vi "StartEqualization.vi"(8 "error in (no error)":errorcluster, 11 "reference in":refnum<class "niMmWave_Transceiver.lvclass">) -> (0 "error out":errorcluster, 2 "channel":T1, 3 "reference out":refnum<class "niMmWave_Transceiver.lvclass">)   [LabVIEW 2019, in "niMmWave_Transceiver.lvclass"]
doc: "Starts generating calibration pulse and prepares RX for acquisition"
uses:
  niMmWave_Transceiver.lvclass
  C:/Barkhausen mmWave radar/Development/LV/Barkhausen mmWave hardware control/Host/SubVIs/mmWave instrument_class/mmWave instrument.lvclass
  mmWave instrument_class/Instrument state.ctl
  Low-level/TypeDefs/TX FPGA Reference.ctl
  Low-level/TypeDefs/TX trigger config.ctl
  FPGA/SubVIs/Utility/FPGA driver trigger source.ctl
  FPGA/SubVIs/Utility/FPGA driver trigger destination.ctl
  <vilib>/Analysis/4window.llb/windowTd.ctl
  <vilib>/Analysis/1siggen.llb/Ramp Pattern by Samples.vi
  <vilib>/Analysis/2dsp.llb/Complex FFT.vi
  <vilib>/Analysis/baseanly.llb/Mean (DBL).vi
  <vilib>/Utility/error.llb/Error Cluster From Error Code.vi
  <vilib>/rvi/errors/niLvFpgaAdjustHostInterfaceError.vi
  <vilib>/measure/mascope.llb/Amplitude and Levels 1 chan.vi
  <vilib>/Analysis/0measdsp.llb/Scaled Time Domain Window (CDB).vi
  <vilib>/Analysis/6fits.llb/1D B-Spline Fit.vi
  <vilib>/rvi/interface/nirviReadWriteControl/nirviReadWriteControl.xnode
  NiFpgaLv.dll
  <vilib>/rvi/interface/Simulation/niFpgaSimulationCallBeginRW.vi
  FPGA/SubVIs/Utility/FPGA Utility.lvlib
  mmWave HW Control/mmWave HW Control.lvlib
  <vilib>/Analysis/NI_AALBase.lvlib
  <vilib>/Analysis/NI_AALPro.lvlib
  mmWave instrument_class/mmWave instrument.lvclass
  <vilib>/measure/NI_MAPro.lvlib
panel:
  out "S/N":dbl
  out "lo":dbl[](array[numeric])
  out "hi":dbl[](array[numeric])
  out "amp":dbl[](array[numeric])
  out "magnitude":T2(graph)
  out "phase":T2(graph)
  out "Waveform Graph - Dark":dbl[][](graph)
  out "phase raw":cluster{"Ramp Pattern":dbl[], dbl[]}[](graph)
  out "magnitude raw":cluster{"Ramp Pattern":dbl[], dbl[]}[](graph)
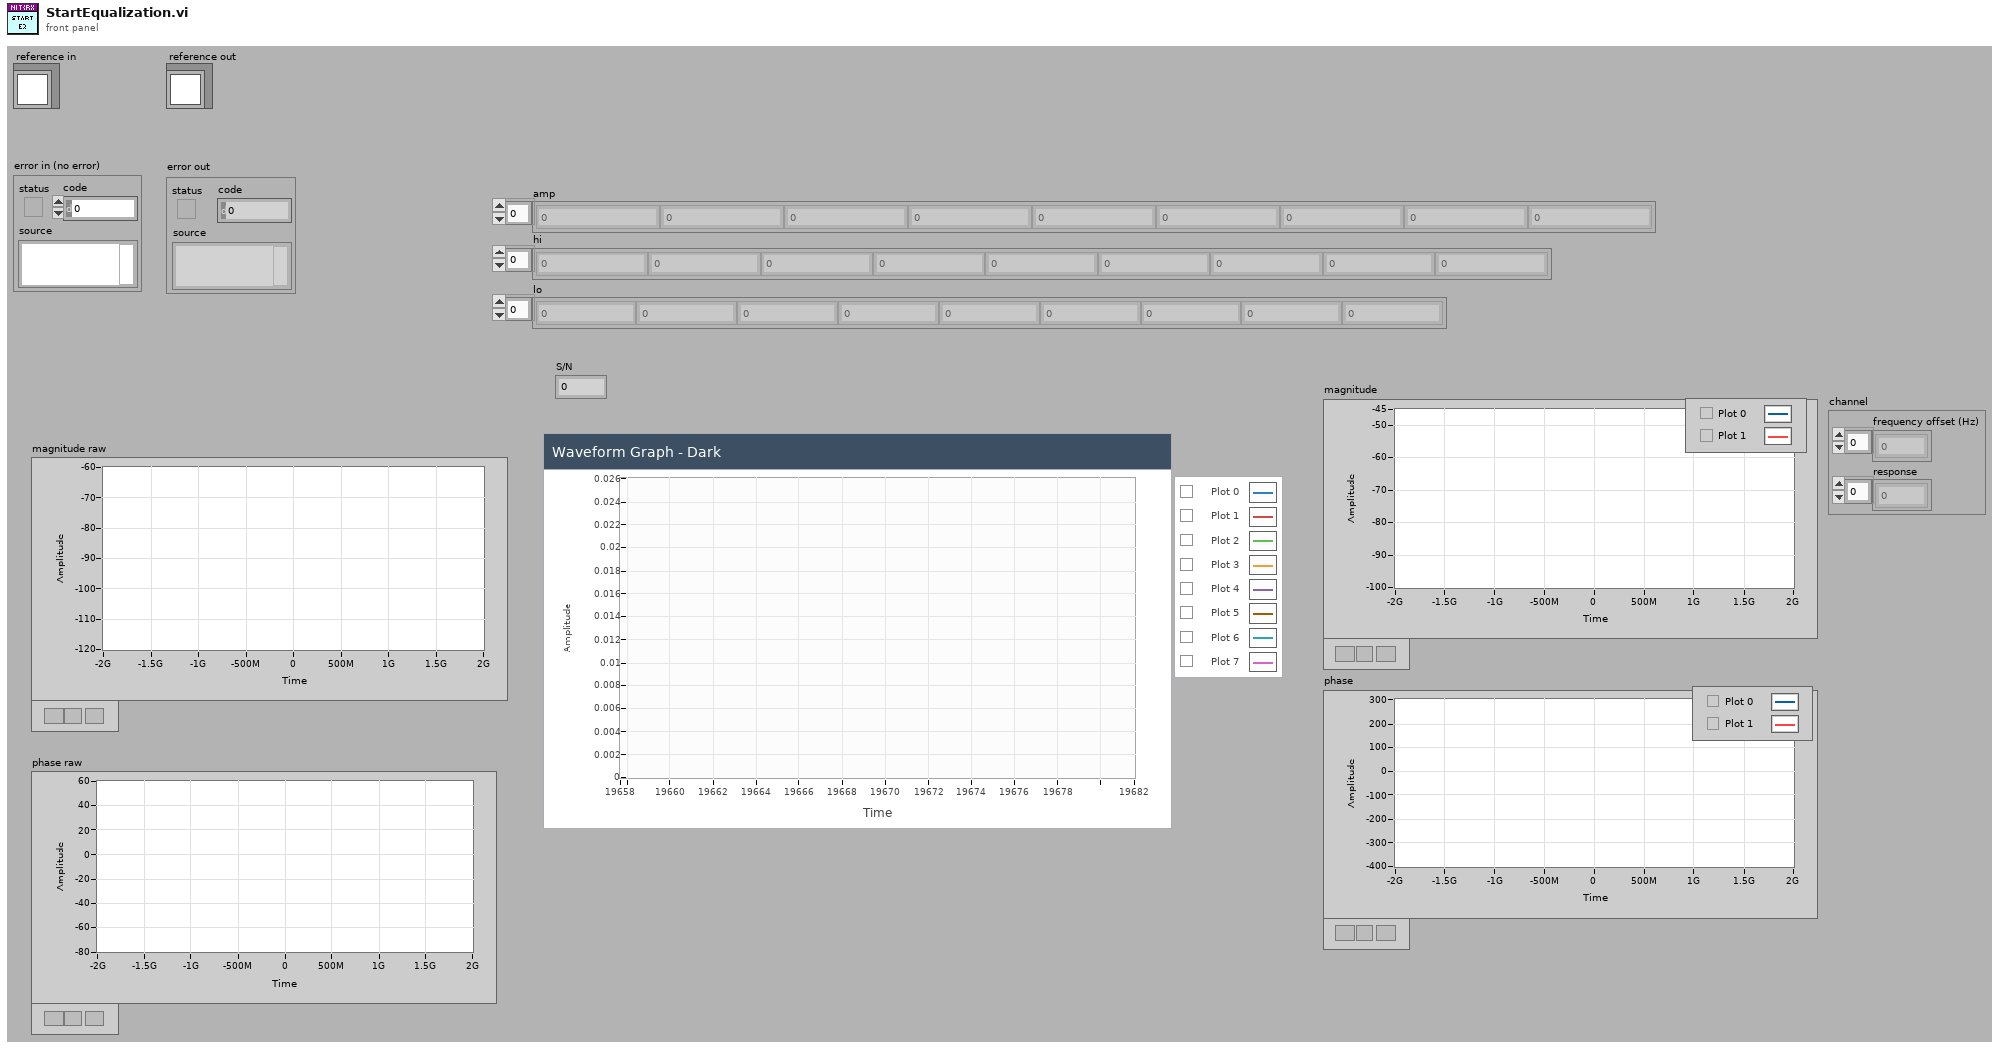
[diagram p1: front panel]
types:
  T1 = cluster{"frequency offset (Hz)":dbl[], "response":cdb[]}
  T2 = cluster{"Ramp Pattern":dbl[], "Best BSpline Fit Y":dbl[]}[]
  T3 = cluster{"frequency":u32, "gain":fxp<+/-,18,1>, "width":u8}
  T4 = typedef "mmWave instrument.lvclass/Instrument state.ctl" = enum16{"Off", "Initialization", "Configuration", "Running", "Calibration"}
  T5 = typedef "TX trigger config.ctl" = cluster{"delay":dbl, "trig source":T6, "PXI src":i32, "export":T7, "PXI dest":i32}
  T6 = typedef "FPGA Utility.lvlib/FPGA driver trigger source.ctl" = enum16{"Use Tclk", "PXI_Trig", "Aurora RX trig"}
  T7 = typedef "FPGA Utility.lvlib/FPGA driver trigger destination.ctl" = enum16{"None", "Source trig", "Synced trig", "Delayed sync"}
  T8 = enum16{"Pass Through", "Tone", "Pulse", "Disable"}
  T9 = typedef "TX FPGA Reference.ctl" = refnum<k20>
  T10 = typedef "niMmWave_Transceiver.lvclass/ObjectAttributesRef.ctl" = refnum<data-value>
  T11 = typedef "niMmWave_Transceiver.lvclass/ObjectAttributes.ctl" = cluster{"session":T12[], "HW.RX resources":T26, "RF config":T27, "RX trigger options":T5, "TX trigger options":T5, "RX samples":i32, "Downloaded Bursts":map{string, T28}, "TX Fs":dbl, "RX Fs":dbl, "burst sequence":string[]}
  T12 = typedef "Session.ctl" = cluster{"3620 session":refnum<queue>, "tx baseband session":T13, "rx baseband session":T21, "tx gain (dB)":dbl, "rx gain (dB)":dbl, "hardware configuration":T22, "gain ranging":T24[], "pxi trigger bus information":T25}
  T13 = typedef "Tx Baseband Session.ctl" = cluster{"3610 session":T14, "7902 reference":T20}
  T14 = typedef "ni3610_and_ni3630_Driver_Lib.lvlib/Main Settings.ctl" = cluster{"VISA resource name":refnum<visa-resource-name>, "Address Space":T15, "window_offset":u32, "register_addresses":T16, "required_MM_fpga_version":cluster{"signature":u32, "hardware":u32, "current revision":u32, "oldest revision":u32}, "CPLD Oldest Compat Version ":cluster{"hardware":u32, "CPLD firmware":u32}, "MM_FPGA_image_location":string, "is_init":bool, "card_type":T17, "DacLmkConfigFileName":string, "AdcLmkConfigFileName":string, "AdcConfigFileName":string, "DacConfigFileName_RevA":string, "DacConfigFileName_RevB":string, "Mulde hardware revision":u8, "bypass DAC PLL\n":bool, "IQ Card Revision":T18, "board capability":T19}
  T15 = typedef "VISA Register Access Address Space.ctl" = u16
  T16 = typedef "ni3610_and_ni3630_Driver_Lib.lvlib/Register Adresses.ctl" = cluster{"MM based Registers":cluster{"Revision":u32, "OldestCompatRev":u32, "signature":u32, "scratch":u32, "LedControl":u32, "BoardHwRev":u32, "BoardControl":u32, "ThermalStatus":u32, "BasebandStatus":u32, "BasebandControl":u32, "BasebandAuxSetup":u32, "BasebandAuxStatus":u32, "LmkSyncOutSetup":u32, " AdcSyncOutSetup":u32, " InjSyncOutSetup":u32, " PxiTrig0OutSetup":u32, " PxiTrig1OutSetup":u32, " PxiTrig2OutSetup":u32, " PxiTrig3OutSetup":u32, " PxiTrig4OutSetup":u32, " PxiTrig5OutSetup":u32, " PxiTrig6OutSetup":u32, " PxiTrig7OutSetup":u32}, "CPLD based Registers":cluster{"SlaveSignature":u32, "SlaveRevision":u32, "SlaveOldestCompatRev":u32, "SlaveScratch":u32, "SlaveSetup":u32, "SlaveStatus":u32, "IDacReg_offset":u32, "LMKRegGrp0_offset":u32, "QDacReg_offset":u32, "BrdTempSensorVal":u32, "TempSensorPowerDown":u32, "GPIOReg_offset":u32, "IAdcReg_offset":u32, "QAdcReg_offset":u32, "LMKRegGrp1_offset":u32, "QadcTempSensorVal":u32, "IadcTempSensorVal":u32, "RevisionReg":u32, "VcxoReg":u32, "CpldStatusReg":u32, "PowerReg":u32, "VBiasEnReg":u32, "ExtRefOeReg":u32, "QdacCtrlReg":u32, "QdacStatusReg":u32, "IdacCtrlReg":u32, "IdacStatusReg":u32, "QdacJtagIn":u32, "QdacJtagOut":u32, "IdacJtagIn":u32, "IdacJtagOut":u32, "IqDcSetupReg":u32, "QadcStatusReg":u32, "IadcStatusReg":u32, "BrdSetupReg":u32, "IqDcRevisionReg":u32, "PllStatusReg":u32, "EndpointScratchReg":u32, "AdcSyncCfgReg":u32, "IqCardOpampReg":u32}, "CPLD Register Offset":u32, "MM  Register Offset":u32, " PxiTrig0OutSetup":u32}
  T17 = typedef "ni3610_and_ni3630_Driver_Lib.lvlib/Base Card Type.ctl" = enum16{"unspecified", "ADC", "DAC"}
  T18 = typedef "ni3610_and_ni3630_Driver_Lib.lvlib/IQ Card Revision.ctl" = enum16{"RevA", "RevB", "RevC", "RevD"}
  T19 = typedef "ni3610_and_ni3630_Driver_Lib.lvlib/Board Capability.ctl" = cluster{"baseband sync":enum16{"no baseband sync", "baseband sync"}}
  T20 = typedef "Blank FPGA Reference.ctl" = refnum<k20>
  T21 = typedef "Rx Baseband Session.ctl" = cluster{"3630 session":T14, "7902 reference":T20}
  T22 = typedef "Hardware Configuration.ctl" = cluster{"direction":T23, "baseband only":bool}
  T23 = typedef "Direction.ctl" = enum16{"Transceiver", "Receiver", "Transmitter"}
  T24 = typedef "Gain Ranging.ctl" = cluster{"gain ranging active scope":string, "gain ranging stream session":refnum<k20>}
  T25 = typedef "PXI Trigger Bus Info.ctl" = cluster{"chassis resource name":refnum<visa-resource-name>, "7902R (TX)":i16, "3610 (TX)":i16, "3620 (IF)":i16, "3630 (RX)":i16, "7902R (RX)":i16}
  T26 = typedef "mmWave HW Control.lvlib/HW TXRX resources cluster.ctl" = cluster{"TX_DAC":refnum<visa-resource-name>, "TX_FPGA":tag, "IF":tag, "RX_ADC":refnum<visa-resource-name>, "RX_FPGA":tag}
  T27 = typedef "mmWave HW Control.lvlib/HW TXRX RF config cluster.ctl" = cluster{"TX.Frequency":dbl, "TX.Gain":dbl, "TX.mmWave adapter":string, "RX.Frequency":dbl, "RX.Gain":dbl, "RX.mmWave adapter":string}
  T28 = typedef "niMmWave_Transceiver.lvclass/BurstInfo.ctl" = cluster{"starting addr":u32, "end addr":u32}
  T29 = cluster{"generation select":enum16{"Pass Through", "Tone", "Pulse", "Disable"}, "tone parameters":cluster{"frequency":fxp<+/-,48,0>, "gain":fxp<+/-,18,1>}, "pulse parameters":cluster{"frequency":u32, "gain":fxp<+/-,18,1>, "width":u8}}
  T30 = typedef "Constants.ctl" = cluster{"data clock rate (Hz)":dbl, "sample rate (Hz)":dbl, "sample rate selector string":string, "default tx bitfile path":path, "default rx bitfile path":path, "default proc bitfile path":path}
  T31 = typedef "NI_AALPro.lvlib/windowTd.ctl" = u32
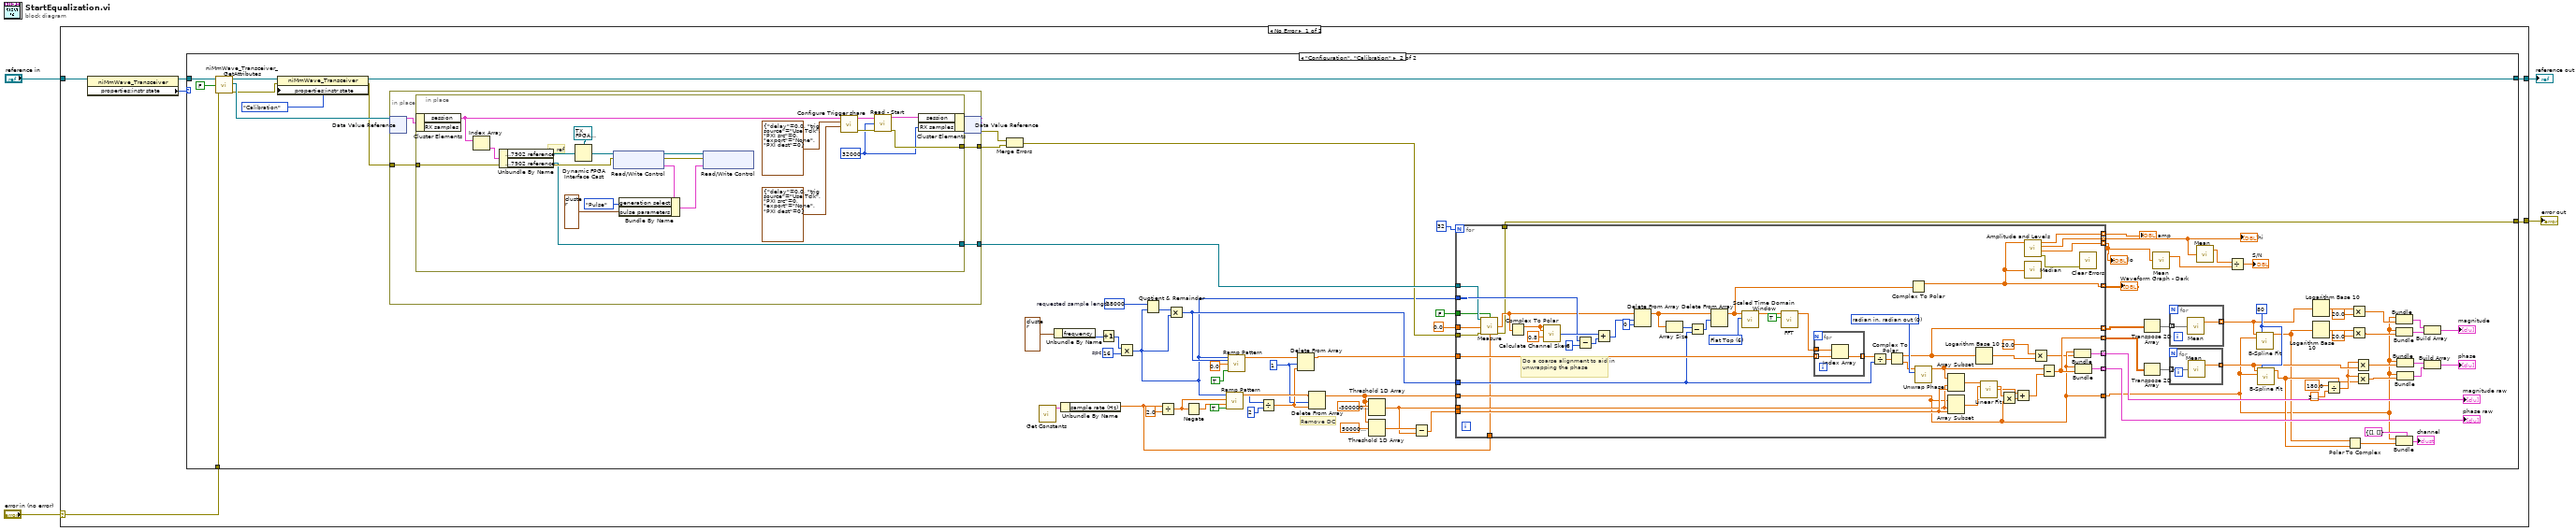
[diagram p0: block diagram]
diagram:
  n1 = case shown="No Error" "error in (no error)" {
    selector: "error in (no error)" -> [w10 w180]
    tunnel: [w6 w180] -> w3
    tunnel: [w7 w179] -> w1
    tunnel: "reference in" -> [w9 w179]
    frame No Error {
      n2 = property class="niMmWave_Transceiver"(reference=w9) -> (reference out=w8:refnum<class "niMmWave_Transceiver.lvclass">, "properties:instr state"=w5:T4)  [unwired: 1 in, 1 out]
      n3 = case shown="\"Configuration\", \"Calibration\"" w5 {
        tunnel: w10 -> [_ w95]
        tunnel: w8 -> [w11 w93]
        tunnel: [w11 w84] -> w7
        tunnel: [_ w78] -> w6
        frame "Off", Default {
        }
        frame "Configuration", "Calibration" {
          w28 = 28000  # requested sample length
          w30 = 1 ("length")
          w27 = u32 16  # spc
          w69 = 80 ("# of control points")
          # "Remove DC"
          n4 = call "niMmWave_Transceiver_GetAttributes.vi"("error in (no error)"=w95, "return data? (T)"=FALSE, "reference in"=w93) -> ("error out"=w47:errorcluster, "attributes ref"=w92:T10, "reference out"=w91:refnum<class "niMmWave_Transceiver.lvclass">)  [unwired: 5 in, 1 out]
          n5 = property class="niMmWave_Transceiver"(reference=w91, error in=w47, "properties:instr state"=Instrument_state."Calibration" ("instr state")) -> (reference out=w84:refnum<class "niMmWave_Transceiver.lvclass">, error out=w46:errorcluster)
          n6 = in-place {
            in-place-border: w46 -> [w156]
            in-place-border: [w155] -> w90
            in-place-border: [w154] -> w82
            n7 = in-place-dvr #1(w92) -> (w158:T11)  [unwired: 1 out]
            n8 = in-place {
              in-place-border: w156 -> [w163]
              in-place-border: [w162] -> w155
              in-place-border: [w160] -> w154
              w161 = u32 32000 ("number of samples")
              # "tx ref"
              n9 = in-place-cluster #2(w158) -> ("session"=w169:T12[])  [unwired: 1 out]
              n10 = Index Array(array=w169) -> (element=w178:T12)  [unwired: 1 in]
              n11 = Unbundle By Name(w178) -> ("tx baseband session.7902 reference"=w177:T20, "rx baseband session.7902 reference"=w160:T20)
              n12 = Dynamic FPGA Interface Cast(Session In=T9 refnum ("Refnum in"), Type=w177) -> (Session Out=w176:T9)
              n13 = xnode "Read/Write Control"("FPGA VI Reference In"=w176, "error in"=w163) -> ("FPGA VI Reference Out"=w175:T9, "error out"=w174:errorcluster, "cal.generation"=w171:T29)
              n14 = Bundle By Name(cluster=w171, "generation select"=T8."Pulse", "pulse parameters"=T3 {"frequency"=10, "gain"=0.5, "width"=1}) -> (w159:T29)
              n15 = xnode "Read/Write Control"("FPGA VI Reference In"=w175, "error in"=w174, "cal.generation"=w159) -> ()  [unwired: 2 out]
              n16 = call "Configure Trigger share.vi"("RX trigger options"=T5 {"delay"=0.0, "trig source"=enum."Use Tclk", "PXI src"=0, "export"=enum."None", "PXI dest"=0} ("TX trigger options"), "TX trigger options"=T5 {"delay"=0.0, "trig source"=enum."Use Tclk", "PXI src"=0, "export"=enum."None", "PXI dest"=0}, "session in"=w169) -> ("error out"=w165:errorcluster, "session out"=w166:T12[])  [unwired: 5 in, 2 out]
              n17 = call "Read - Start.vi"("session in"=w166, "number of samples"=w161, "error in"=w165) -> ("session out"=w164:T12[], "error out"=w162:errorcluster)  [unwired: 11 in]
              n18 = in-place-cluster #2("session"=w164, "RX samples"=w161) -> (w157:T11)
            }
            n19 = in-place-dvr #1(w157) -> (w89:errorcluster)  [unwired: 1 out]
          }
          n20 = Merge Errors(w89, w90) -> (w79:errorcluster)
          n21 = call "Get Constants.vi"() -> ("constants"=w45:T30)  [unwired: 15 in]
          n22 = Unbundle By Name(T3 {"frequency"=10, "gain"=0.5, "width"=1} ("pulse parameters")) -> ("frequency"=w19:u32)
          n23 = Unbundle By Name(w45) -> ("sample rate (Hz)"=w18:dbl)
          n24 = Increment(x=w19) -> (x+1=w37:u32)
          n25 = Multiply(x=w37, y=w27) -> (x*y=w21:u32)
          n26 = Quotient & Remainder(x=w28, y=w21) -> (floor(x/y)=w43:u32)  [unwired: 1 out]
          n27 = Divide(x=w18, y=2.0) -> (x/y=w39:dbl)
          n28 = Multiply(x=w43, y=w21) -> (x*y=w22:u32)
          n29 = Negate(x=w39) -> (-x=w38:dbl)
          n30 = call-poly <vilib>:"Ramp Pattern.vi"("exclude end?"=TRUE, "start"=w38, "end"=w39, "samples"=w21) -> ("Ramp Pattern"=w42:dbl[])  [unwired: 6 in, 1 out]
          n31 = call-poly <vilib>:"Ramp Pattern.vi"("exclude end?"=TRUE, "start"=0.0, "end"=w22, "samples"=w21) -> ("Ramp Pattern"=w40:dbl[])  [unwired: 6 in, 1 out]
          n32 = Divide(x=w21, y=2) -> (x/y=w41:dbl)
          n33 = Delete From Array(array=w40, length=w30, index=w41) -> (array with subset deleted=w24:dbl[])  [unwired: 1 out]
          n34 = Delete From Array(array=w42, length=w30, index=w41) -> (array with subset deleted=w23:dbl[])  [unwired: 1 out]
          n35 = Threshold 1D Array(2:500000000.0 ("threshold y"), 3:w23) -> (0:w44:dbl)  [unwired: 1 in]
          n36 = Threshold 1D Array(2:-500000000.0 ("threshold y"), 3:w23) -> (0:w25:dbl)  [unwired: 1 in]
          n37 = Subtract(x=w44, y=w25) -> (x-y=w26:dbl)
          n38 = for {
            N: 32 -> [_]
            tunnel: [w128] -> w50 mode=indexing
            tunnel: w23 -> [w122]
            tunnel: w21 -> [w131]
            tunnel: [w122] -> w49
            tunnel: [w116] -> w51 mode=indexing
            tunnel: w24 -> [w140]
            tunnel: [w146] -> w88 mode=indexing
            tunnel: [w141] -> w87 mode=indexing
            tunnel: w22 -> [w130]
            tunnel: w26 -> [w124]
            tunnel: w25 -> [w123]
            tunnel: [w104] -> w85 mode=indexing
            tunnel: w82 -> [w111]
            tunnel: FALSE ("calculate measurements") -> [w110]
            tunnel: 0.0 ("frequency (Hz)") -> [w109]
            tunnel: w79 -> [w108]
            tunnel: w18 -> [w107]
            tunnel: [w105] -> w78
            tunnel: [w102] -> w17 mode=indexing
            tunnel: [w101] -> w16 mode=indexing
            tunnel: [w100] -> w15 mode=indexing
            w129 = T31 6 items=["Rectangle"=0, "Hanning"=1, "Hamming"=2, "Blackman-Harris"=3, "Exact Blackman"=4, "Blackman"=5, "Flat Top"=6, "4 Term B-Harris "=7, "7 Term B-Harris"=8, "Low Sidelobe"=9, "Blackman Nuttall"=11, "Triangle"=30, "Bartlett-Hanning"=31, "Bohman"=32, "Parzen"=33, "Welch"=34, "Kaiser"=60, "Dolph-Chebyshev"=61, "Gaussian"=62] ("window")
            w142 = 0 items=["radian in, radian out", "radian in, degree out", "degree in, degree out", "degree in, radian out"] ("phase unit")
            # "Do a coarse alignment to aid in unwrapping the phase"
            n39 = call "Measure.vi"("rx fpga reference in"=w111, "calculate measurements"=w110, "frequency (Hz)"=w109, "error in"=w108, "IQ rate"=w107) -> ("raw data"=w106:cdb[], "error out"=w105:errorcluster)  [unwired: 7 in, 2 out]
            n40 = Complex To Polar(r * e^(i*theta)=w106) -> (r=w133:dbl[])  [unwired: 1 out]
            n41 = call "Calculate Channel Skew.vi"("channel 1"=w133, "channel 2"=w133, "threshold"=0.8) -> ("falling edge index"=w138:i32)  [unwired: 10 in, 2 out]
            n42 = Subtract(x=w131, y=8) -> (x-y=w136:u32)
            n43 = Add(x=w138, y=w136) -> (x+y=w134:u32)
            n44 = Delete From Array(array=w106, length=w134, index=0) -> (array with subset deleted=w132:cdb[])  [unwired: 1 out]
            n45 = Array Size(array=w132) -> (size(s)=w149:i32)
            n46 = Subtract(x=w149, y=w130) -> (x-y=w148:u32)
            n47 = Delete From Array(array=w132, length=w148) -> (array with subset deleted=w112:cdb[])  [unwired: 1 in, 1 out]
            n48 = call-poly <vilib>:"Scaled Time Domain Window.vi"("window"=w129, "X"=w112) -> ("Windowed X"=w147:cdb[])  [unwired: 7 in, 2 out]
            n49 = call-poly <vilib>:"FFT.vi"("shift?"=TRUE, "X"=w147) -> ("FFT {X}"=w143:cdb[])  [unwired: 8 in, 1 out]
            n50 = for {
              tunnel: w140 -> [w153] mode=indexing
              tunnel: w143 -> [w152]
              tunnel: [w151] -> w145 mode=indexing
              n51 = Index Array(array=w152, index=w153) -> (element=w151:cdb)
            }
            n52 = Divide(x=w145, y=w130) -> (x/y=w144:cdb[])
            n53 = Complex To Polar(r * e^(i*theta)=w144) -> (r=w116:dbl[], theta=w117:dbl[])
            n54 = Complex To Polar(r * e^(i*theta)=w112) -> (r=w104:dbl[])  [unwired: 1 out]
            n55 = call <vilib>:"Unwrap Phase.vi"("phase unit"=w142, "Phase"=w117) -> ("Unwrapped Phase"=w127:dbl[])  [unwired: 8 in, 1 out]
            n56 = Array Subset(array=w127, index=w123, length=w124) -> (w126:dbl[])
            n57 = Array Subset(array=w122, index=w123, length=w124) -> (w125:dbl[])
            n58 = Logarithm Base 10(1:w116) -> (0:w115:dbl[])
            n59 = call <vilib>:"Linear Fit.vi"("Y"=w126, "X"=w125) -> ("slope"=w121:dbl, "intercept"=w119:dbl)  [unwired: 9 in, 3 out]
            n60 = Multiply(x=w121, y=w122) -> (x*y=w120:dbl[])
            n61 = Add(x=w119, y=w120) -> (x+y=w118:dbl[])
            n62 = call-poly <vilib>:"Amplitude and Levels.vi"("signal in"=w104) -> ("error out"=w103:errorcluster, "low state level"=w100:dbl, "high state level"=w101:dbl, "amplitude"=w102:dbl)  [unwired: 7 in]
            n63 = call <vilib>:"Median.vi"("X"=w104) -> ()  [unwired: 2 out]
            n64 = Multiply(x=20.0, y=w115) -> (x*y=w113:dbl[])
            n65 = Subtract(x=w127, y=w118) -> (x-y=w128:dbl[])
            n66 = Bundle("Ramp Pattern"=w122, w113) -> (w146:cluster{"Ramp Pattern":dbl[], dbl[]})  [unwired: 1 in]
            n67 = Bundle("Ramp Pattern"=w122, w128) -> (w141:cluster{"Ramp Pattern":dbl[], dbl[]})  [unwired: 1 in]
            n68 = call <vilib>:"Clear Errors.vi"("error in (no error)"=w103) -> ()  [unwired: 5 in, 2 out]
          }
          "magnitude raw" <- w88
          "phase raw" <- w87
          "Waveform Graph - Dark" <- w85
          "amp" <- w17
          "hi" <- w16
          "lo" <- w15
          n69 = Transpose 2D Array(2D array=w51) -> (transposed array=w76:dbl[][])
          n70 = Transpose 2D Array(2D array=w50) -> (transposed array=w77:dbl[][])
          n71 = call-poly <vilib>:"Mean.vi"("X"=w15) -> ("mean"=w13:dbl)  [unwired: 1 out]
          n72 = for {
            tunnel: w77 -> [w97] mode=indexing
            tunnel: [w96] -> w64 mode=indexing
            n73 = call-poly <vilib>:"Mean.vi"("X"=w97) -> ("mean"=w96:dbl)  [unwired: 1 out]
          }
          n74 = for {
            tunnel: w76 -> [w99] mode=indexing
            tunnel: [w98] -> w58 mode=indexing
            n75 = call-poly <vilib>:"Mean.vi"("X"=w99) -> ("mean"=w98:dbl)  [unwired: 1 out]
          }
          n76 = call-poly <vilib>:"Mean.vi"("X"=w16) -> ("mean"=w14:dbl)  [unwired: 1 out]
          n77 = Divide(x=w14, y=w13) -> (x/y=→"S/N":dbl)
          n78 = call-poly <vilib>:"B-Spline Fit.vi"("Y"=w58, "# of control points"=w69, "X"=w49) -> ("Best BSpline Fit Y"=w53:dbl[])  [unwired: 9 in, 3 out]
          n79 = call-poly <vilib>:"B-Spline Fit.vi"("Y"=w64, "# of control points"=w69, "X"=w49) -> ("Best BSpline Fit Y"=w61:dbl[])  [unwired: 9 in, 3 out]
          n80 = Logarithm Base 10(1:w58) -> (0:w57:dbl[])
          n81 = Logarithm Base 10(1:w53) -> (0:w54:dbl[])
          n82 = Divide(x=180.0, y=3.141592653589793) -> (x/y=w62:dbl)
          n83 = Polar To Complex(1:w61, 2:w53) -> (0:w68:cdb[])
          n84 = Multiply(x=w57, y=20.0) -> (x*y=w56:dbl[])
          n85 = Multiply(x=w54, y=20.0) -> (x*y=w52:dbl[])
          n86 = Multiply(x=w62, y=w64) -> (x*y=w63:dbl[])
          n87 = Multiply(x=w62, y=w61) -> (x*y=w60:dbl[])
          n88 = Bundle("Ramp Pattern"=w49, w56) -> (w75:cluster{"Ramp Pattern":dbl[], dbl[]})  [unwired: 1 in]
          n89 = Bundle("Ramp Pattern"=w49, w52) -> (w74:cluster{"Ramp Pattern":dbl[], dbl[]})  [unwired: 1 in]
          n90 = Bundle(cluster=T1 {"frequency offset (Hz)"=[], "response"=[]} ("channel 2"), "frequency offset (Hz)"=w49, "response"=w68) -> (→"channel":T1)
          n91 = Bundle("Ramp Pattern"=w49, w63) -> (w72:cluster{"Ramp Pattern":dbl[], dbl[]})  [unwired: 1 in]
          n92 = Bundle("Ramp Pattern"=w49, w60) -> (w71:cluster{"Ramp Pattern":dbl[], dbl[]})  [unwired: 1 in]
          n93 = Build Array(w75, w74) -> (→"magnitude":cluster{"Ramp Pattern":dbl[], dbl[]}[])
          n94 = Build Array(w72, w71) -> (→"phase":cluster{"Ramp Pattern":dbl[], dbl[]}[])
        }
      }
    }
    frame Error {
    }
  }
  "error out" <- w3
  "reference out" <- w1
